vi "StartStream.vi"(2 "error in (no error)":errorcluster, 3 "OphirRef In":T1) -> (0 "error out":errorcluster, 1 "OphirRef Out":T1)   [LabVIEW 2012]
uses:
  TypeDefs/OphirRef.ctl
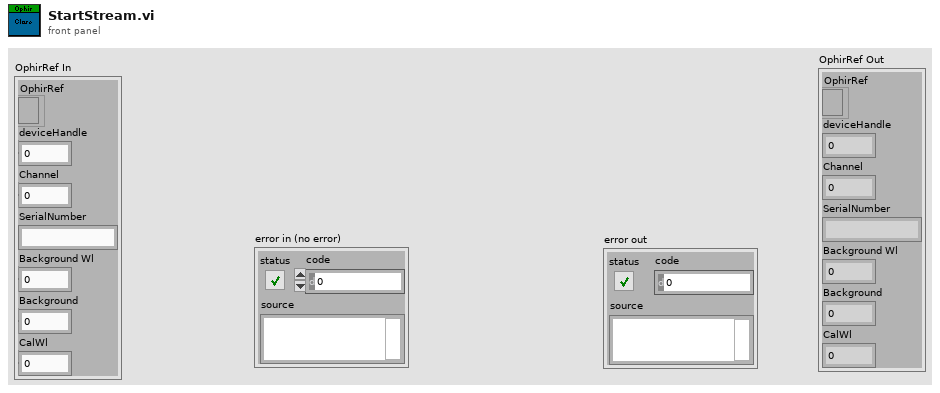
[diagram p1: front panel]
types:
  T1 = typedef "OphirRef.ctl" = cluster{"OphirRef":refnum<k7>, "deviceHandle":i32, "Channel":i32, "SerialNumber":string, "Background Wl":dbl, "Background":dbl, "CalWl":dbl}
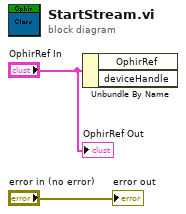
[diagram p0: block diagram]
diagram:
  n1 = Unbundle By Name("OphirRef In") -> ()  [unwired: 2 out]
  "OphirRef Out" <- "OphirRef In"
  "error out" <- "error in (no error)"
